vi "Action Name.vi"(8 "error in (no error)":errorcluster, 11 "Filter by Is Send In":refnum<class "Filter by Is Broadcast.lvclass">) -> (0 "error out":errorcluster, 2 "Action Name":string, 3 "Filter by Is Send Out":refnum<class "Filter by Is Broadcast.lvclass">)   [LabVIEW 2020, in "Filter by Is Broadcast.lvclass"]
uses:
  Filter by Is Broadcast.lvclass
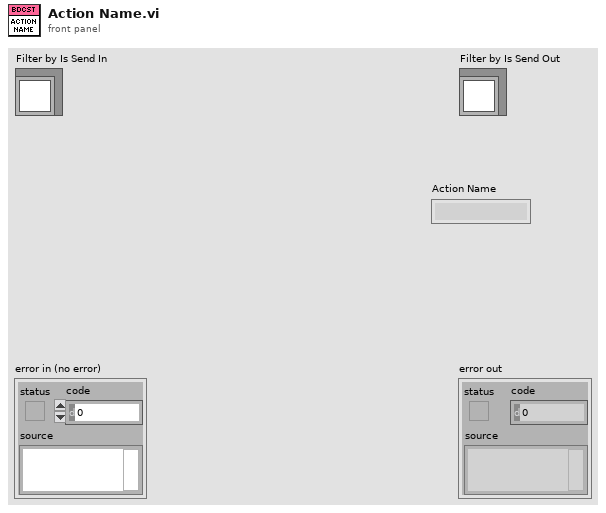
[diagram p1: front panel]
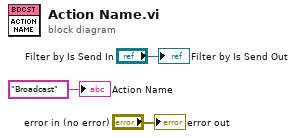
[diagram p0: block diagram]
diagram:
  "error out" <- "error in (no error)"
  "Filter by Is Send Out" <- "Filter by Is Send In"
  "Action Name" <- "Broadcast" ("Action Name")
